vi "DDMs_low_initialize.vi"(7 "Measurement":T1(ring), 8 "error in (no error)":errorcluster, 10 "Device":T2(ring), 11 "VISA resource name":refnum<visa-resource-name>) -> (0 "error out":errorcluster, 3 "VISA resource name out":refnum<visa-resource-name>)   [LabVIEW 2020, in "DMMsData.lvclass"]
uses:
  DMMsData.lvclass
  istr.lib/ADCMT7451A_ADC/Public/Configure/Configure DC Volts.vi
  <instrlib>/Agilent 34401/Agilent 34401.lvlib
  istr.lib/ADCMT7351_ADC/ADCMT7351_ADC.lvlib
  istr.lib/ADCMT7451A_ADC/ADCMT7451_ADC.lvlib
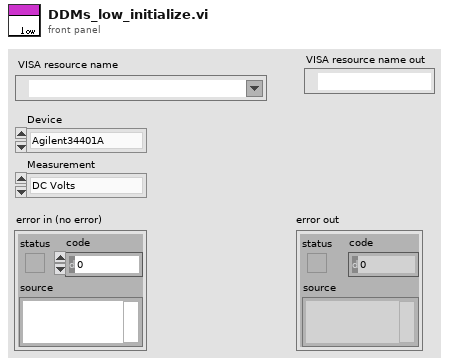
[diagram p1: front panel]
types:
  T1 = enum16{"DC Volts", "DC Currents", "2-Wire Resistance", "4-Wire Resistance"}
  T2 = enum16{"Agilent34401A", "ADCMT7351", "HP3478A", "ADCMT7451"}
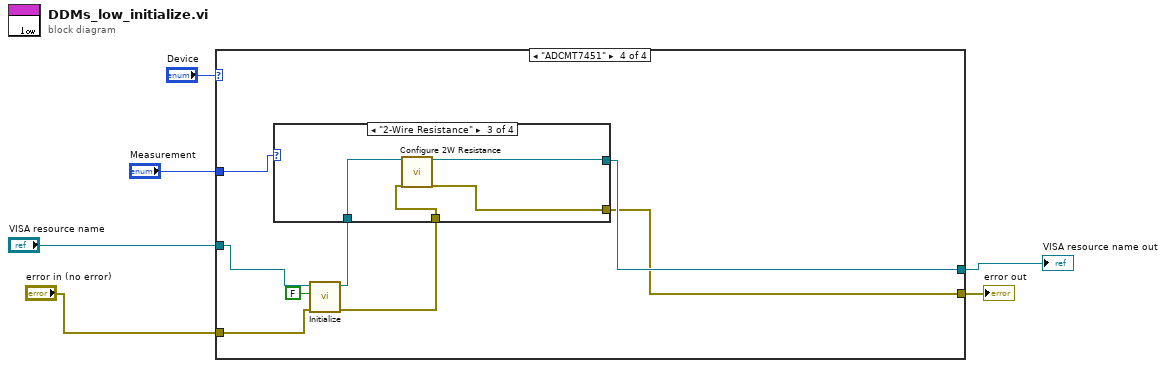
[diagram p0: block diagram]
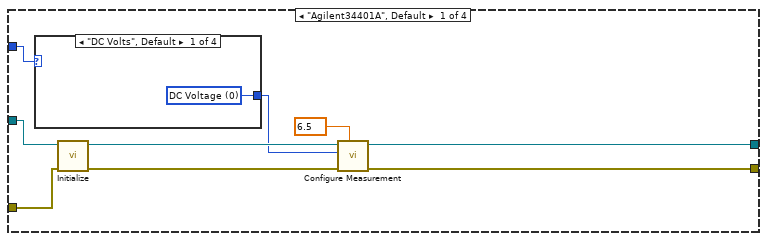
[diagram p2: hidden frame]
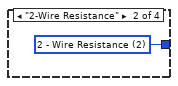
[diagram p3: hidden frame]
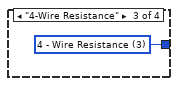
[diagram p4: hidden frame]
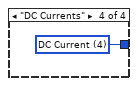
[diagram p5: hidden frame]
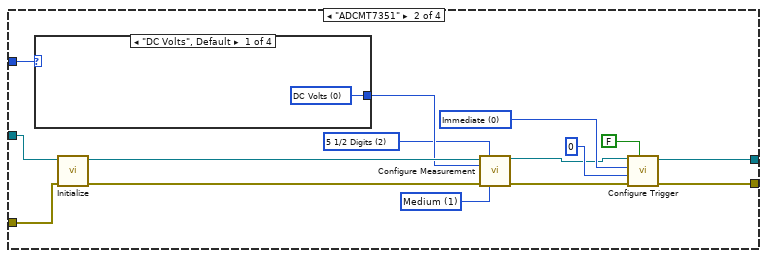
[diagram p6: hidden frame]
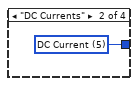
[diagram p7: hidden frame]
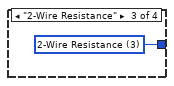
[diagram p8: hidden frame]
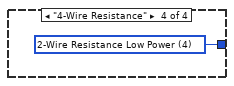
[diagram p9: hidden frame]
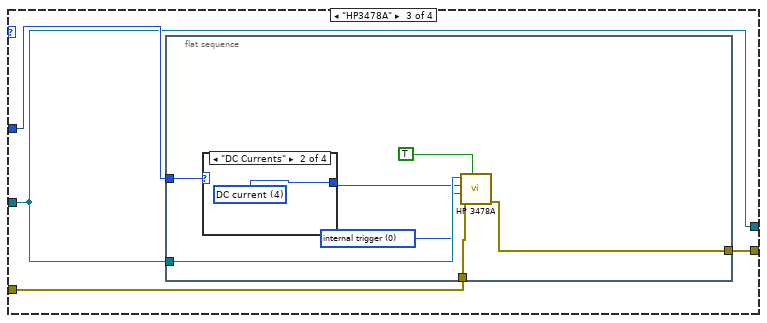
[diagram p10: hidden frame]
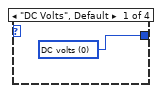
[diagram p11: hidden frame]
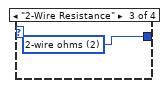
[diagram p12: hidden frame]
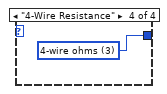
[diagram p13: hidden frame]
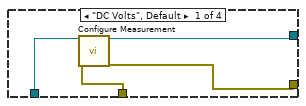
[diagram p14: hidden frame]
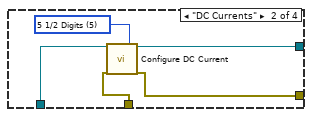
[diagram p15: hidden frame]
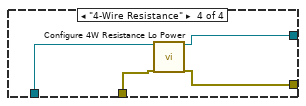
[diagram p16: hidden frame]
diagram:
  n1 = case shown="\"ADCMT7451\"" "Device" {
    tunnel: "VISA resource name" -> [w15 w34 w41 w60]
    tunnel: "Measurement" -> [w14 w31 w42 w61]
    tunnel: [w9 w22 w41 w55] -> w3
    tunnel: [w8 w24 w39 w54] -> w2
    tunnel: "error in (no error)" -> [w7 w20 w40 w57]
    frame "Agilent34401A", Default {
      w10 = 6.5 items=["4.5"=4.5, "5.5"=5.5, "6.5"=6.5] ("Manual Resolution (5.5 Digits)")
      n2 = case shown="\"DC Volts\", Default" w14 {
        tunnel: [w16 w17 w18 w19] -> w11
        frame "DC Volts", Default {
          w16 = u16 0 items=["DC Voltage", "AC Voltage", "2 - Wire Resistance", "4 - Wire Resistance", "DC Current", "AC Current", "Frequency", "Period", "Continuity", "Diode Checking", "VDC:VDC Ratio", "Temperature", "Capacitance"] ("Function (0: DC Voltage)")
        }
        frame "2-Wire Resistance" {
          w17 = u16 2 items=["DC Voltage", "AC Voltage", "2 - Wire Resistance", "4 - Wire Resistance", "DC Current", "AC Current", "Frequency", "Period", "Continuity", "Diode Checking", "VDC:VDC Ratio", "Temperature", "Capacitance"] ("Function (0: DC Voltage)")
        }
        frame "4-Wire Resistance" {
          w18 = u16 3 items=["DC Voltage", "AC Voltage", "2 - Wire Resistance", "4 - Wire Resistance", "DC Current", "AC Current", "Frequency", "Period", "Continuity", "Diode Checking", "VDC:VDC Ratio", "Temperature", "Capacitance"] ("Function (0: DC Voltage)")
        }
        frame "DC Currents" {
          w19 = u16 4 items=["DC Voltage", "AC Voltage", "2 - Wire Resistance", "4 - Wire Resistance", "DC Current", "AC Current", "Frequency", "Period", "Continuity", "Diode Checking", "VDC:VDC Ratio", "Temperature", "Capacitance"] ("Function (0: DC Voltage)")
        }
      }
      n3 = call <instrlib>:"Initialize.vi"("error in (no error)"=w7, "VISA resource name"=w15) -> ("error out"=w12:errorcluster, "VISA resource name out"=w13:refnum<visa-resource-name>)  [unwired: 8 in]
      n4 = call <instrlib>:"Configure Measurement.vi"("Manual Resolution (5.5 Digits)"=w10, "error in (no error)"=w12, "Function (0: DC Voltage)"=w11, "VISA resource name"=w13) -> ("error out"=w8:errorcluster, "VISA resource name out"=w9:refnum<visa-resource-name>)  [unwired: 6 in]
    }
    frame "ADCMT7351" {
      w27 = u16 0 items=["Immediate", "Manual", "External", "Bus"] ("Trigger Source")
      w28 = u16 1 items=["Fast", "Medium", "Slow 1", "Slow 2"] ("Sampling Rate (3: Slow 2)")
      w29 = u16 2 items=["3 1/2 Digits", "4 1/2 Digits", "5 1/2 Digits"] ("Digits (2: 5 1/2)")
      n5 = case shown="\"DC Volts\", Default" w31 {
        tunnel: [w35 w36 w37 w38] -> w30
        frame "DC Volts", Default {
          w35 = u16 0 items=["DC Volts", "AC Volts", "AC+DC Volts", "2-Wire Resistance", "2-Wire Resistance Low Power", "DC Current", "AC Current", "AC+DC Current", "Diode", "Continuity", "Frequency"] ("Function (0: DC Volts)")
        }
        frame "DC Currents" {
          w36 = u16 5 items=["DC Volts", "AC Volts", "AC+DC Volts", "2-Wire Resistance", "2-Wire Resistance Low Power", "DC Current", "AC Current", "AC+DC Current", "Diode", "Continuity", "Frequency"] ("Function (0: DC Volts)")
        }
        frame "2-Wire Resistance" {
          w37 = u16 3 items=["DC Volts", "AC Volts", "AC+DC Volts", "2-Wire Resistance", "2-Wire Resistance Low Power", "DC Current", "AC Current", "AC+DC Current", "Diode", "Continuity", "Frequency"] ("Function (0: DC Volts)")
        }
        frame "4-Wire Resistance" {
          w38 = u16 4 items=["DC Volts", "AC Volts", "AC+DC Volts", "2-Wire Resistance", "2-Wire Resistance Low Power", "DC Current", "AC Current", "AC+DC Current", "Diode", "Continuity", "Frequency"] ("Function (0: DC Volts)")
        }
      }
      n6 = call <instrlib>:"Initialize.vi"("error in (no error)"=w20, "VISA resource name"=w34) -> ("error out"=w32:errorcluster, "VISA resource name out"=w33:refnum<visa-resource-name>)  [unwired: 8 in]
      n7 = call <instrlib>:"Configure Measurement.vi"("VISA resource name"=w33, "Digits (2: 5 1/2)"=w29, "Function (0: DC Volts)"=w30, "error in (no error)"=w32, "Sampling Rate (3: Slow 2)"=w28) -> ("VISA resource name out"=w23:refnum<visa-resource-name>, "error out"=w25:errorcluster)  [unwired: 9 in]
      n8 = call "Configure Trigger.vi"("Enable Trigger Delay (Enable)"=FALSE, "error in (no error)"=w25, "Trigger Delay (0 second)"=0, "Trigger Source (0: Immediate)"=w27, "VISA resource name"=w23) -> ("error out"=w24:errorcluster, "VISA resource name out"=w22:refnum<visa-resource-name>)  [unwired: 5 in]
    }
    frame "HP3478A" {
      n9 = flat-sequence {
        tunnel: w42 -> [w49]
        tunnel: w41 -> [w48]
        tunnel: w40 -> [w44]
        tunnel: [w43] -> w39
        frame #0 {
          w46 = i16 0 items=["internal trigger", "single trigger", "external trigger", "trigger hold", "fast trigger"] ("trigger mode")
          n10 = case shown="\"DC Currents\"" w49 {
            tunnel: [w50 w51 w52 w53] -> w47
            frame "DC Volts", Default {
              w50 = i16 0 items=["DC volts", "AC volts", "2-wire ohms", "4-wire ohms", "DC current", "AC current", "extended ohms"] ("measurement")
            }
            frame "DC Currents" {
              w51 = i16 4 items=["DC volts", "AC volts", "2-wire ohms", "4-wire ohms", "DC current", "AC current", "extended ohms"] ("measurement")
            }
            frame "2-Wire Resistance" {
              w52 = i16 2 items=["DC volts", "AC volts", "2-wire ohms", "4-wire ohms", "DC current", "AC current", "extended ohms"] ("measurement")
            }
            frame "4-Wire Resistance" {
              w53 = i16 3 items=["DC volts", "AC volts", "2-wire ohms", "4-wire ohms", "DC current", "AC current", "extended ohms"] ("measurement")
            }
          }
          n11 = call "HP 3478A.vi"("autorange"=TRUE, "error in"=w44, "trigger mode"=w46, "measurement"=w47, "VISA resource name"=w48) -> ("error out"=w43:errorcluster)  [unwired: 3 in, 1 out]
        }
      }
    }
    frame "ADCMT7451" {
      n12 = call <instrlib>:"Initialize.vi"("error in (no error)"=w57, "ID Query (True)"=FALSE, "VISA resource name"=w60) -> ("error out"=w56:errorcluster, "VISA resource name out"=w59:refnum<visa-resource-name>)  [unwired: 7 in]
      n13 = case shown="\"2-Wire Resistance\"" w61 {
        tunnel: w59 -> [w65 w70 w74 w78]
        tunnel: w56 -> [w64 w69 w73 w77]
        tunnel: [w63 w68 w72 w75] -> w54
        tunnel: [w62 w66 w71 w76] -> w55
        frame "DC Volts", Default {
          n14 = call-poly <instrlib>:"Configure Measurement.vi"("VISA resource name"=w65, "error in (no error)"=w64) -> ("VISA resource name out"=w62:refnum<visa-resource-name>, "error out"=w63:errorcluster)  [unwired: 16 in]
        }
        frame "DC Currents" {
          w67 = u16 5 items=["3 1/2 Digits"=3, "4 1/2 Digits"=4, "5 1/2 Digits"=5] ("Digits (5: 5 1/2)")
          n15 = call "Configure DC Current.vi"("VISA resource name"=w70, "error in (no error)"=w69, "Digits (5: 5 1/2)"=w67) -> ("VISA resource name out"=w66:refnum<visa-resource-name>, "error out"=w68:errorcluster)  [unwired: 15 in]
        }
        frame "2-Wire Resistance" {
          n16 = call "Configure 2W Resistance.vi"("VISA resource name"=w74, "error in (no error)"=w73) -> ("VISA resource name out"=w71:refnum<visa-resource-name>, "error out"=w72:errorcluster)  [unwired: 16 in]
        }
        frame "4-Wire Resistance" {
          n17 = call "Configure 4W Resistance Lo Power.vi"("VISA resource name"=w78, "error in (no error)"=w77) -> ("VISA resource name out"=w76:refnum<visa-resource-name>, "error out"=w75:errorcluster)  [unwired: 16 in]
        }
      }
    }
  }
  "VISA resource name out" <- w3
  "error out" <- w2
